vi "PWM.vi"() -> ()   [LabVIEW 2015]
doc: "This VI uses a PWM Out (subVI).vi to generate a pulse train on DIO 0 according to the Low Period and High Period controls. It then uses PWM In (subVI).vi to measure DIO 1 and report the measured Low Period and High Period.\n\nHardware Connection Required - Use a wire to physically connect DIO0 to DIO1."
uses:
  <vilib>/Platform/TimedLoop/XDataNode/timing_clust.ctl
  <vilib>/Platform/TimedLoop/XDataNode/nitl_modes.ctl
  <vilib>/Platform/TimedLoop/XDataNode/wakeup.ctl
  <vilib>/rvi/Emulation/niFpgaGetClockAttributes.vi
  <vilib>/rvi/Emulation/niFpgaSctlEmulationGetInTimedLoop.vi
  <vilib>/rvi/Emulation/niFpgaEmulationReportErrorSimple.vi
  <vilib>/rvi/eio/common/nirviEmuTemplateMethod_errors.vi
  <vilib>/rvi/Emulation/niFpgaCriticalErrorInLSC.vi
  <vilib>/eio/EIONode/EIONode.xnode
  <vilib>/Platform/TimedLoop/XDataNode/XDataNode.xnode
  <vilib>/Platform/TimedLoop/XDataNode/XDNodeRunTimeDep.lvlib
panel:
  in  "Stop Input":bool
  out "Output":bool
  in  "Stop Output":bool
  out "High Period (ms)":u32=500
  out "Low Period (ms)":u32=500
  in  "High Period (ms)":u16=500
  in  "Low Period (ms)":u16=500
  # "This VI uses a PWM Out (subVI).vi to generate a pulse train on DIO 0 according to the \nLow Period and High Period controls.  It then uses PWM In (subVI).vi to measure DIO 1 \nand report the measured Low Period and High Period.\nHardware Connection Required - Use a wire to physically connect DIO0 to DIO1."
  # "Output"
  # "Measure"
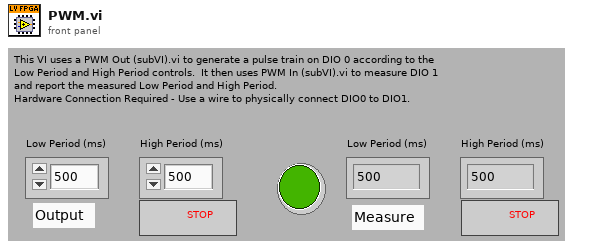
[diagram p1: front panel]
types:
  T1 = typedef "XDNodeRunTimeDep.lvlib/timing_clust.ctl" = cluster{"Expected End [f-1]":u64, "Actual End [f-1]":u64, "Finished Late? [f-1]":bool, "Expected End [i-1]":u64, "Actual End [i-1]":u64, "Finished Late? [i-1]":bool, "Expected Start [i]":u64, "Actual Start [i]":u64, "Expected Start [f]":u64, "Actual Start [f]":u64, "Source Name":string, "Structure Name":string, "Period":i64, "Deadline":i64, "Offset":i64, "Start":i64, "Priority":i32, "Timeout":i32, "Mode":T2, "Wakeup Reason":T3, "Error":errorcluster, "Source Type":string, "Secondary Source Type":string, "Global End Time":u64, "Global Start Time":u64, "Frame Duration":u64, "Iteration Duration":u64, "Assigned CPU":i32, "I/O Scan Engine Mode":u32}
  T2 = typedef "XDNodeRunTimeDep.lvlib/nitl_modes.ctl" = enum32{"No Change", "Process missed periods, maintain original phase", "Discard missed periods, maintain original phase", "Process missed periods, ignore original phase", "Discard missed periods, ignore original phase"}
  T3 = typedef "XDNodeRunTimeDep.lvlib/wakeup.ctl" = enum32{"Normal", "Aborted", "Asynchronous wakeup", "Timing source error", "Timed loop error", "Timeout"}
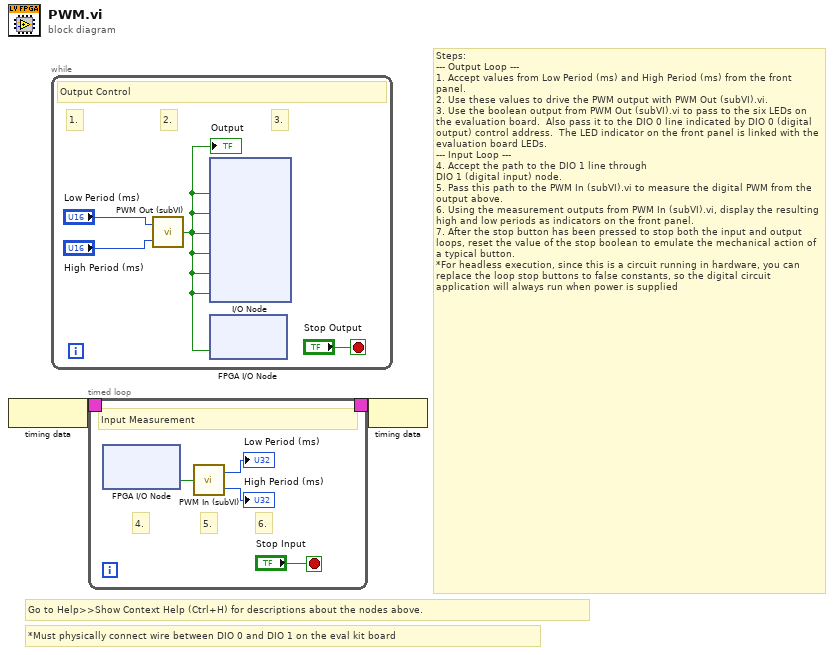
[diagram p0: block diagram]
diagram:
  # "*Must physically connect wire between DIO 0 and DIO 1 on the eval kit board"
  # "Go to Help>>Show Context Help (Ctrl+H) for descriptions about the nodes above."
  # "Steps:\n--- Output Loop ---\n1. Accept values from Low Period (ms) and High Period (ms) from the front panel.\n2. Use these values to drive the PWM output with PWM Out (subVI).vi.\n3. Use the boolean output from PWM Out (subVI).vi to pass to the six LEDs on the evaluation board.  Also pass it to the DIO 0 line indicated by DIO 0 (digital output) control address.  The LED indicator on the front panel is linked with the evaluation board LEDs.\n--- Input Loop ---\n4. Accept the path to the DIO 1 line through \nDIO 1 (digital input) node.\n5. Pass this path to the PWM In (subVI).vi to measure the digital PWM from the output above.\n6. Using the measurement outputs from PWM In (subVI).vi, display the resulting high and low periods as indicators on the front panel.\n7. After the stop button has been pressed to stop both the input and output loops, reset the value of the stop boolean to emulate the mechanical action of a typical button.\n*For headless execution, since this is a circuit running in hardware, you can replace the loop stop buttons to false constants, so the digital circuit application will always run when power is supplied"
  n1 = node-c288() -> (w2:T1)
  n2 = while {
    stop <- "Stop Output" stop-if-true
    # "3."
    # "2."
    # "1."
    # "Output Control"
    n3 = call "PWM Out (subVI).vi"("High Pulse"="High Period (ms)", "Low Pulse"="Low Period (ms)") -> ("PWM Output"=w3:bool)
    "Output" <- w3
    n4 = xnode "I/O Node"("LED 1"=w3, "LED 2"=w3, "LED 3"=w3, "LED 4"=w3, "LED 5"=w3, "LED 6"=w3) -> ()  [unwired: 6 in, 6 out]
    n5 = xnode "FPGA I/O Node"("DIO0"=w3) -> ()  [unwired: 1 in, 1 out]
  }
  n6 = timed-loop {
    timing: w2 -> [_]
    timing-out: [_] -> w1
    stop <- "Stop Input" stop-if-true
    # "6."
    # "5."
    # "4."
    # "Input Measurement"
    n7 = xnode "FPGA I/O Node"() -> ("DIO1"=w7:bool)  [unwired: 1 in, 1 out]
    n8 = call "PWM In (subVI).vi"("PWM Input"=w7) -> ("Low Period"=→"Low Period (ms)":u32, "High Period"=→"High Period (ms)":u32)
  }
  n9 = node-c288(w1) -> ()
